vi "IDs to Names.vi"(10 "IDs":T1) -> (2 "Names":string[](array[string]))   [LabVIEW 2019, in "Tool Data.lvclass"]
uses:
  Tool Data.lvclass
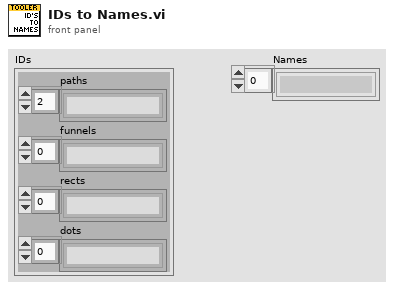
[diagram p1: front panel]
types:
  T1 = cluster{"paths":string[], "funnels":string[], "rects":string[], "dots":string[]}
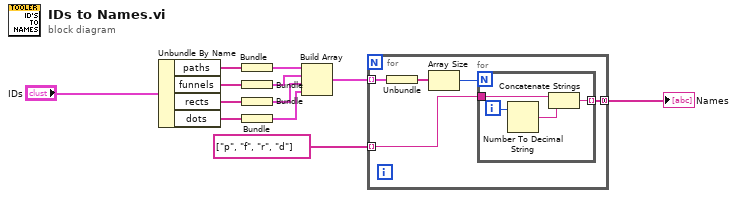
[diagram p0: block diagram]
diagram:
  n1 = Unbundle By Name("IDs") -> ("paths"=w11:string[], "funnels"=w10:string[], "rects"=w9:string[], "dots"=w8:string[])
  n2 = Bundle("paths"=w11) -> (w7:cluster{"paths":string[]})  [unwired: 1 in]
  n3 = Bundle("funnels"=w10) -> (w6:cluster{"funnels":string[]})  [unwired: 1 in]
  n4 = Bundle("rects"=w9) -> (w5:cluster{"rects":string[]})  [unwired: 1 in]
  n5 = Bundle("dots"=w8) -> (w4:cluster{"dots":string[]})  [unwired: 1 in]
  n6 = Build Array(w7, w6, w5, w4) -> (w2:cluster{"dots":string[]}[])
  n7 = for {
    tunnel: string[] ["p", "f", "r", "d"] -> [w14] mode=indexing
    tunnel: w2 -> [w17] mode=indexing
    tunnel: [w13] -> w1 mode=concatenating
    n8 = Unbundle(w17) -> ("dots"=w16:string[])
    n9 = Array Size(array=w16) -> (size(s)=w15:i32)
    n10 = for {
      N: w15 -> [_]
      tunnel: w14 -> [w20]
      tunnel: [w18] -> w13 mode=indexing
      i -> [w21]
      n11 = Number To Decimal String(number=w21) -> (decimal integer string=w19:string)  [unwired: 1 in]
      n12 = Concatenate Strings(w20, w19) -> (w18:string)
    }
  }
  "Names" <- w1
